vi "Create Sine Wave (SubVI).vi"(8 "error in (no error)":errorcluster, 10 "sampling info":cluster{"Fs":dbl, "#s":dbl}={"Fs"=1000.0, "#s"=1000.0}, 11 "Sine Waveform Settings":T1(array[cluster])=[{"Frequency (Hz)"=1000.0, "Amplitude (V)"=4.0, "Offset (V)"=0.0, "Phase (deg)"=0.0}, {"Frequency (Hz)"=100.0, "Amplitude (V)"=3.0, "Offset (V)"=0.0, "Phase (deg)"=0.0}]) -> (0 "error out":errorcluster, 2 "FXP Sinewave":fxp<+/-,24,4>[](array[numeric]), 3 "Voltage Output Waveform":waveform(dbl)[](array[waveform]))   [LabVIEW 2021]
doc: "This VI creates a sine wave based on the sampling information and sine waveform settings controls. It outputs the sine wave created as a Waveform and Fixed Point (24,4) data-type."
uses:
  <vilib>/measure/NI_MABase.lvlib
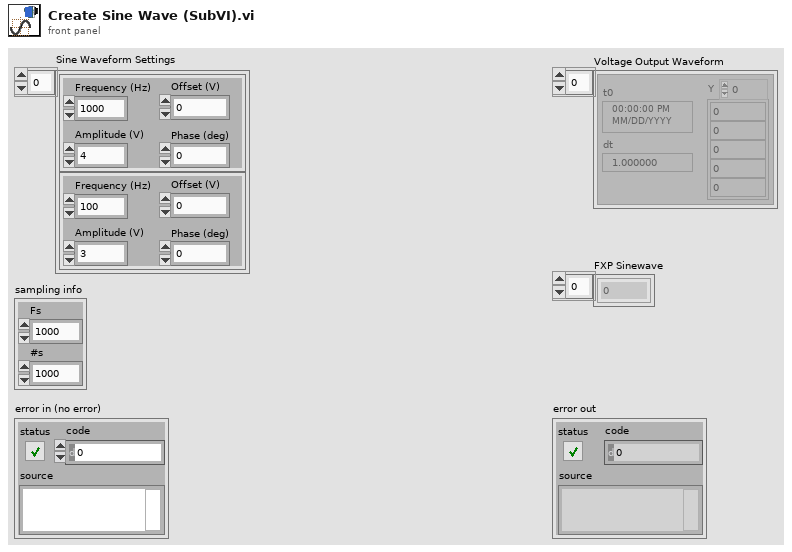
[diagram p1: front panel]
types:
  T1 = cluster{"Frequency (Hz)":dbl, "Amplitude (V)":dbl, "Offset (V)":dbl, "Phase (deg)":dbl}[]
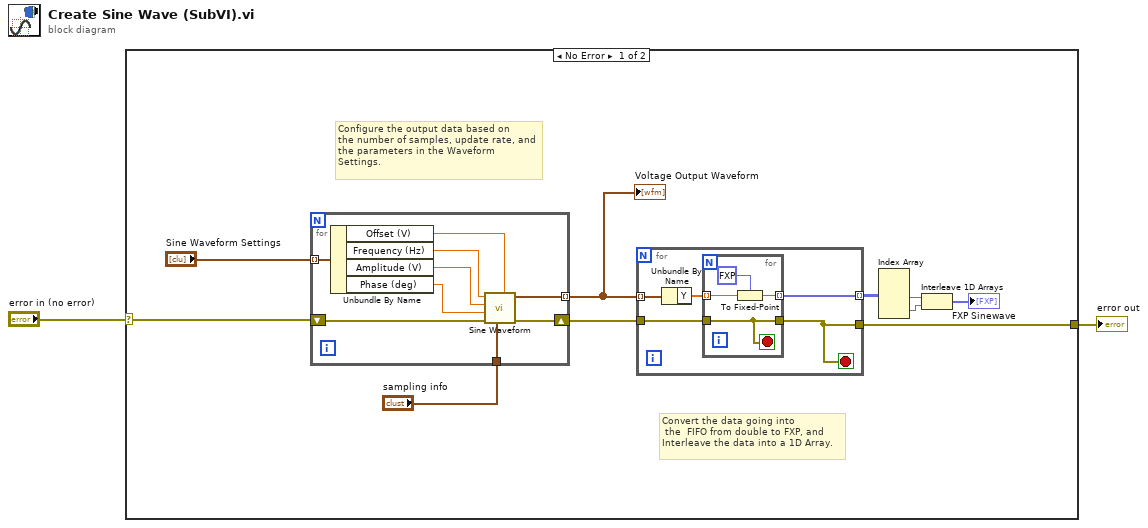
[diagram p0: block diagram]
diagram:
  n1 = case shown="No Error" "error in (no error)" {
    selector: "error in (no error)" -> [w6 w31]
    tunnel: [w4 w31] -> w1
    frame No Error {
      # "Convert the data going into\n the  FIFO from double to FXP, and\nInterleave the data into a 1D Array."
      # "Configure the output data based on\nthe number of samples, update rate, and the parameters in the Waveform Settings."
      n2 = for {
        tunnel: "sampling info" -> [w30]
        shift-right: [w29] -> w5
        shift-left: w6 -> [w28]
        tunnel: "Sine Waveform Settings" -> [w27] mode=indexing
        tunnel: [w22] -> w11 mode=indexing
        n3 = Unbundle By Name(w27) -> ("Offset (V)"=w23:dbl, "Frequency (Hz)"=w24:dbl, "Amplitude (V)"=w25:dbl, "Phase (deg)"=w26:dbl)
        n4 = call <vilib>:"Sine Waveform.vi"("offset"=w23, "sampling info"=w30, "error in (no error)"=w28, "phase"=w26, "amplitude"=w25, "frequency"=w24) -> ("error out"=w29:errorcluster, "signal out"=w22:waveform(dbl))  [unwired: 4 in]
      }
      "Voltage Output Waveform" <- w11
      n5 = for {
        tunnel: w11 -> [w16] mode=indexing
        tunnel: [w15] -> w10 mode=indexing
        tunnel: w5 -> [w14]
        tunnel: [w13] -> w4
        stop <- w13 stop-if-true
        n6 = Unbundle By Name(w16) -> ("Y"=w17:dbl[])
        n7 = for {
          tunnel: w17 -> [w21] mode=indexing
          tunnel: [w20] -> w15 mode=indexing
          tunnel: w14 -> [w18]
          tunnel: [w18] -> w13
          stop <- w18 stop-if-true
          n8 = To Fixed-Point(fixed-point type=fxp<+/-,24,4> 0.0, number=w21) -> (fixed-point=w20:fxp<+/-,24,4>)
        }
      }
      n9 = Index Array(array=w10) -> (element #1=w9:fxp<+/-,24,4>[], element #2=w8:fxp<+/-,24,4>[])  [unwired: 4 in]
      n10 = Interleave 1D Arrays(w9, w8) -> (→"FXP Sinewave":fxp<+/-,24,4>[])
    }
    frame Error {
    }
  }
  "error out" <- w1
